vi "OAT Get Order Sequence for Synthesis.vi"(4 "orders to extract":cluster{"orders to extract":dbl[]}[](array[cluster])) -> (1 "order sequence":dbl[](array[numeric]))   [LabVIEW 2017, in "SoundVib_Gabor.lvlib"]
uses:
  <vilib>/addons/Sound and Vibration/Order Analysis/Gabor Order Tracking/SoundVib_Gabor.lvlib
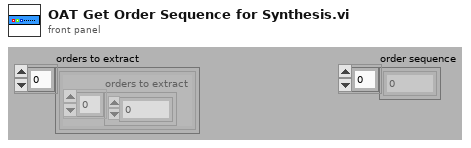
[diagram p1: front panel]
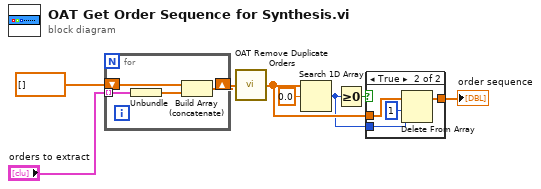
[diagram p0: block diagram]
diagram:
  n1 = for {
    tunnel: "orders to extract" -> [w10] mode=indexing
    shift-right: [w11] -> w7
    shift-left: dbl[] [] ("array in") -> [w12]
    n2 = Unbundle(w10) -> ("orders to extract"=w9:dbl[])
    n3 = Build Array (concatenate)(w12, w9) -> (w11:dbl[])
  }
  n4 = call <vilib>:"OAT Remove Duplicate Orders.vi"("array in"=w7) -> ("array out"=w4:dbl[])
  n5 = Search 1D Array(1D array=w4, element=0.0) -> (index of element=w3:i32)  [unwired: 1 in]
  n6 = Greater Or Equal To 0?(x=w3) -> (x >= 0?=w5:bool)
  n7 = case shown="True" w5 {
    tunnel: w4 -> [w13 w17]
    tunnel: w3 -> [_ w16]
    tunnel: [w13 w14] -> w1
    frame False {
    }
    frame True {
      n8 = Delete From Array(array=w17, length=1, index=w16) -> (array with subset deleted=w14:dbl[])  [unwired: 1 out]
    }
  }
  "order sequence" <- w1
